vi "Wrap Data.vi"(7 "Start Time":timestamp, 8 "error in (no error)":errorcluster, 9 "Data in":refnum<class "Data.lvclass">, 10 "Actor in":refnum<class "Actor.lvclass">, 11 "Response Msg":refnum<class "Response Msg.lvclass">) -> (0 "error out":errorcluster, 1 "Data out":refnum<class "Data.lvclass">, 2 "Actor out":refnum<class "Actor.lvclass">)   [LabVIEW 2020, in "Publisher.lvlib" / "Response Msg.lvclass"]
doc: "The Wrap Data VI allows the Actor and/or message to interact with the data before it is sent or published."
uses:
  Response Msg.lvclass
  PPL/HDH.Actor Framework.Core.Actor.lvlibp/1abvi3w/vi.lib/ActorFramework/Actor/Actor.lvclass
  PPL/HDH.Data.Generic.lvlibp/Data.lvclass
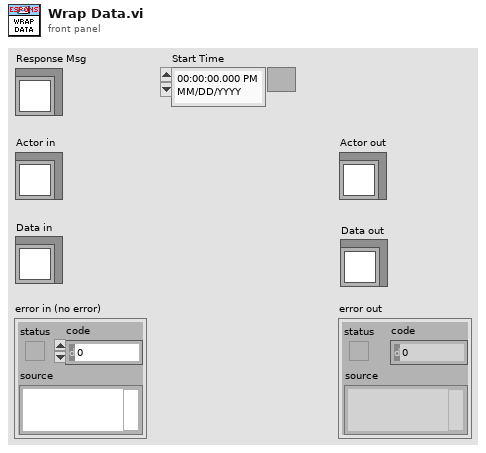
[diagram p1: front panel]
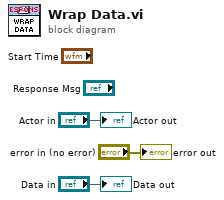
[diagram p0: block diagram]
diagram:
  "error out" <- "error in (no error)"
  "Actor out" <- "Actor in"
  "Data out" <- "Data in"
